vi "Configure Phase Start Stop.vi"(6 "Stop Phase (0 degree)":dbl, 7 "Start Phase (0 degree)":dbl, 8 "error in (no error)":errorcluster, 9 "Port (1)":i32=1, 10 "Channel (1)":i32=1, 11 "VISA resource name":refnum<visa-resource-name>) -> (0 "error out":errorcluster, 3 "VISA resource name out":refnum<visa-resource-name>)   [LabVIEW 2018, in "Keysight PNA Series.lvlib"]
doc: "Configures the start value and stop value of phase sweep."
uses:
  Keysight PNA Series.lvlib
panel:
  # "Note:\nThis VI might need a PNA\nlicense to run properly."
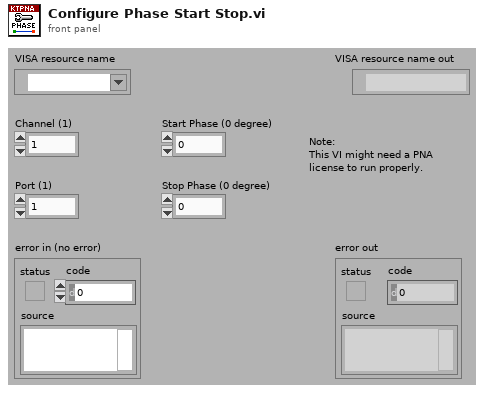
[diagram p1: front panel]
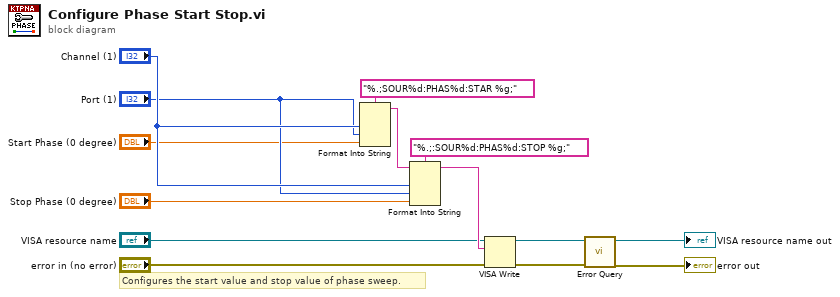
[diagram p0: block diagram]
diagram:
  # "Configures the start value and stop value of phase sweep."
  n1 = Format Into String(format string="%.;SOUR%d:PHAS%d:STAR %g;", "Channel (1)", "Port (1)", "Start Phase (0 degree)") -> (resulting string=w10:string)  [unwired: 2 in, 1 out]
  n2 = Format Into String(format string="%.;:SOUR%d:PHAS%d:STOP %g;", initial string=w10, "Channel (1)", "Port (1)", "Stop Phase (0 degree)") -> (resulting string=w7:string)  [unwired: 1 in, 1 out]
  n3 = VISA Write(VISA resource name="VISA resource name", write buffer=w7, error in (no error)="error in (no error)") -> (VISA resource name out=w4:refnum<visa-resource-name>, error out=w3:errorcluster)  [unwired: 1 out]
  n4 = call "Error Query.vi"("error in (no error)"=w3, "VISA resource name"=w4) -> ("error out"=→"error out":errorcluster, "VISA resource name out"=→"VISA resource name out":refnum<visa-resource-name>)  [unwired: 6 in, 2 out]
